vi "Demo_Trigger_Gen.vi"(5 "0_Stop":bool, 7 "Station No":u32, 8 "Ack":bool[](array[boolean]), 9 "Ack old":bool[](array[boolean]), 10 "Trig":bool[](array[boolean]), 11 "Trig old":bool[](array[boolean])) -> (3 "State to Log":cluster{"State":string, "Station No":string}[](array[cluster]))   [LabVIEW 2017]
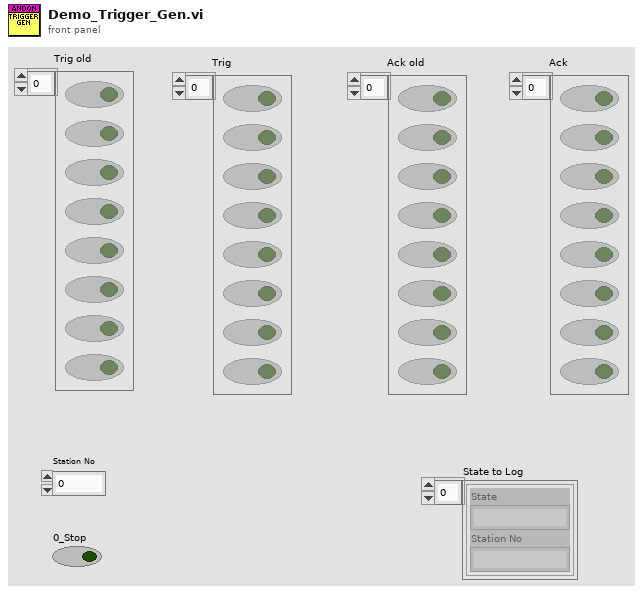
[diagram p1: front panel]
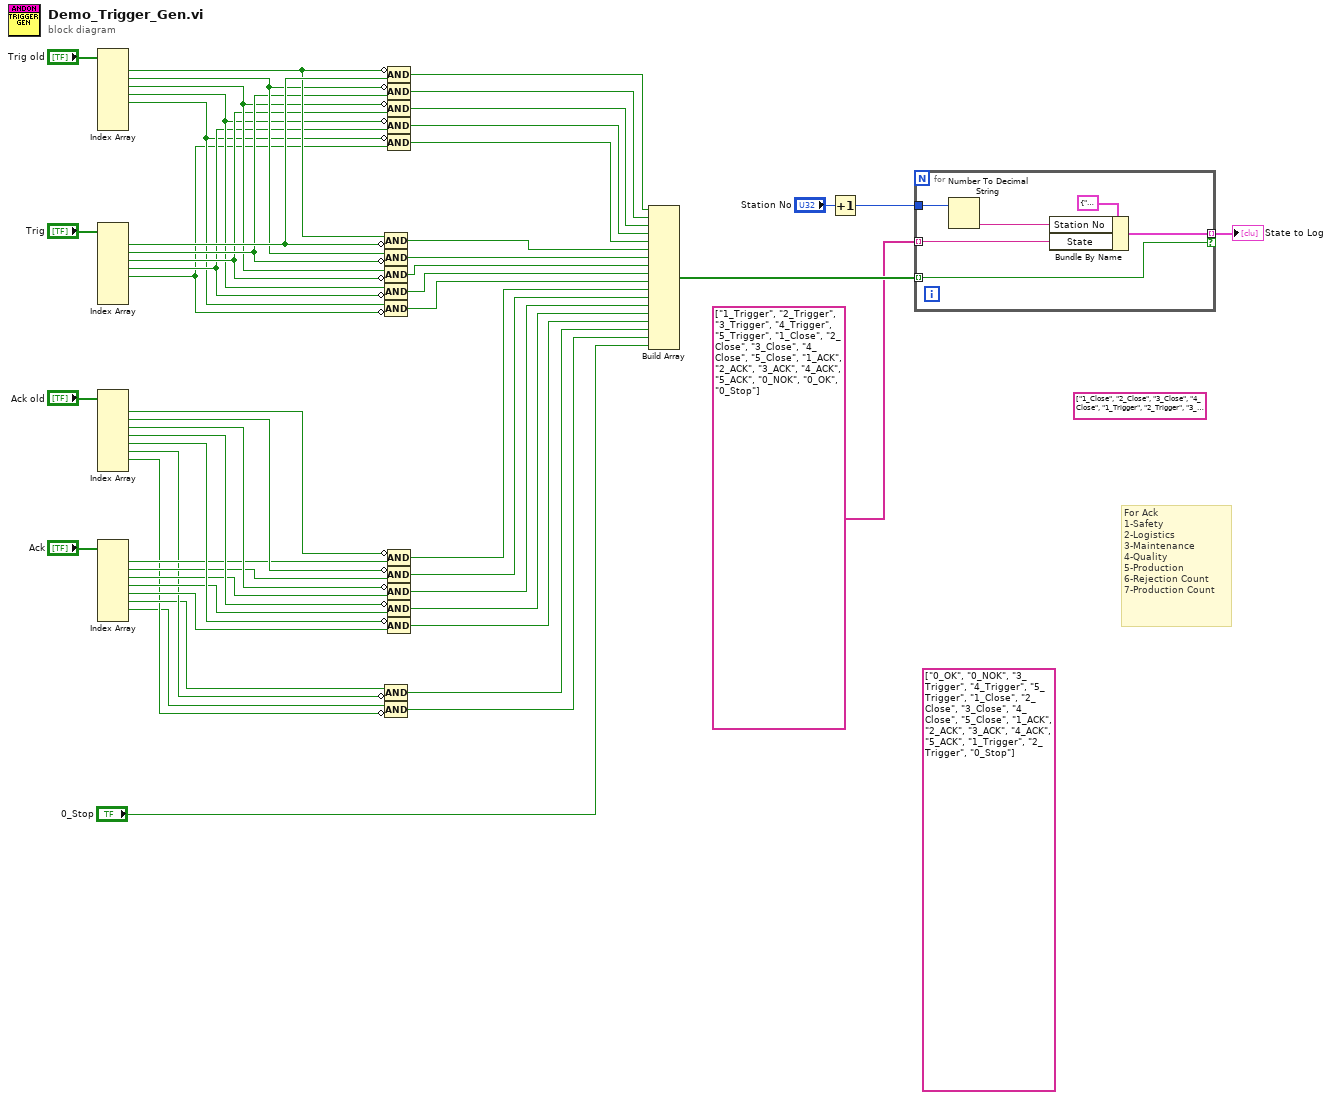
[diagram p0: block diagram]
diagram:
  (unwired) string[] ["1_Close", "2_Close", "3_Close", "4_Close", "1_Trigger", "2_Trigger", "3_Trigger", "4_Trigger", "1_ACK", "2_ACK", "3_ACK", "4_ACK", "0_Stop", "0_OK", "0_NOK"]
  (unwired) string[] ["0_OK", "0_NOK", "3_Trigger", "4_Trigger", "5_Trigger", "1_Close", "2_Close", "3_Close", "4_Close", "5_Close", "1_ACK", "2_ACK", "3_ACK", "4_ACK", "5_ACK", "1_Trigger", "2_Trigger", "0_Stop"]
  # "For Ack\n1-Safety\n2-Logistics\n3-Maintenance\n4-Quality\n5-Production\n6-Rejection Count\n7-Production Count"
  n1 = Index Array(array="Trig old") -> (element #1=w48:bool, element #2=w47:bool, element #3=w45:bool, element #4=w43:bool, element #5=w41:bool)  [unwired: 8 in, 3 out]
  n2 = Index Array(array="Trig") -> (element #1=w49:bool, element #2=w46:bool, element #3=w44:bool, element #4=w42:bool, element #5=w40:bool)  [unwired: 8 in, 3 out]
  n3 = Index Array(array="Ack old") -> (element #1=w31:bool, element #2=w32:bool, element #3=w34:bool, element #4=w36:bool, element #5=w38:bool, element #6=w27:bool, element #7=w15:bool)  [unwired: 8 in, 1 out]
  n4 = Index Array(array="Ack") -> (element #1=w30:bool, element #2=w33:bool, element #3=w35:bool, element #4=w37:bool, element #5=w39:bool, element #6=w26:bool, element #7=w14:bool)  [unwired: 8 in, 1 out]
  n5 = Compound Arithmetic op=AND(w48, invert w49) -> (w20:bool)
  n6 = Compound Arithmetic op=AND(w47, invert w46) -> (w19:bool)
  n7 = Compound Arithmetic op=AND(w45, invert w44) -> (w18:bool)
  n8 = Compound Arithmetic op=AND(w43, invert w42) -> (w17:bool)
  n9 = Compound Arithmetic op=AND(w41, invert w40) -> (w16:bool)
  n10 = Compound Arithmetic op=AND(w26, invert w27) -> (w8:bool)
  n11 = Compound Arithmetic op=AND(w14, invert w15) -> (w7:bool)
  n12 = Compound Arithmetic op=AND(invert w48, w49) -> (w25:bool)
  n13 = Compound Arithmetic op=AND(invert w47, w46) -> (w24:bool)
  n14 = Compound Arithmetic op=AND(invert w45, w44) -> (w23:bool)
  n15 = Compound Arithmetic op=AND(invert w43, w42) -> (w22:bool)
  n16 = Compound Arithmetic op=AND(invert w41, w40) -> (w21:bool)
  n17 = Compound Arithmetic op=AND(invert w31, w30) -> (w13:bool)
  n18 = Compound Arithmetic op=AND(invert w32, w33) -> (w12:bool)
  n19 = Compound Arithmetic op=AND(invert w34, w35) -> (w11:bool)
  n20 = Compound Arithmetic op=AND(invert w36, w37) -> (w10:bool)
  n21 = Compound Arithmetic op=AND(invert w38, w39) -> (w9:bool)
  n22 = Build Array(w25, w24, w23, w22, w21, w20, w19, w18, w17, w16, w13, w12, w11, w10, w9, w8, w7, "0_Stop") -> (w5:bool[])
  n23 = Increment(x="Station No") -> (x+1=w6:u32)
  n24 = for {
    tunnel: w5 -> [w57] mode=indexing
    tunnel: string[] ["1_Trigger", "2_Trigger", "3_Trigger", "4_Trigger", "5_Trigger", "1_Close", "2_Close", "3_Close", "4_Close", "5_Close", "1_ACK", "2_ACK", "3_ACK", "4_ACK", "5_ACK", "0_NOK", "0_OK", "0_Stop"] -> [w55] mode=indexing
    tunnel: [w54] -> w3 mode=indexing if=w57
    tunnel: w6 -> [w53]
    n25 = Number To Decimal String(number=w53) -> (decimal integer string=w52:string)  [unwired: 1 in]
    n26 = Bundle By Name(cluster=cluster{"State":string, "Station No":string} {"State"="", "Station No"=""}, "Station No"=w52, "State"=w55) -> (w54:cluster{"State":string, "Station No":string})
  }
  "State to Log" <- w3
